vi "decode data frame.vi"(11 "字符串":string) -> (3 "EXO message":T1)   [LabVIEW 2016, in "EXO2-Sonde.lvlib"]
uses:
  EXO2-Sonde.lvlib
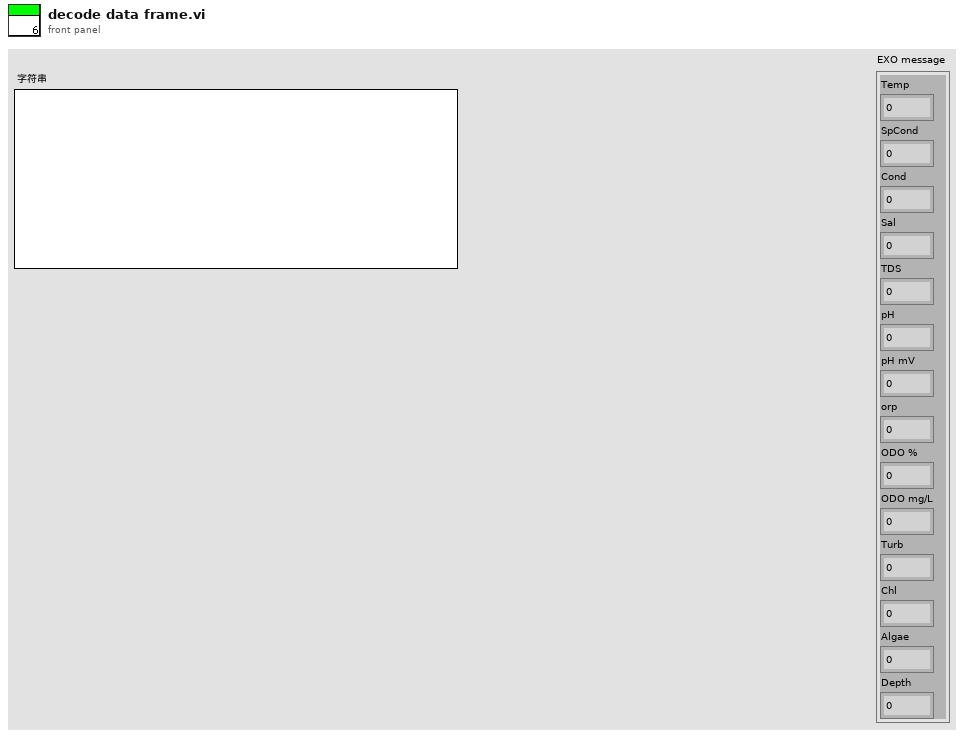
[diagram p1: front panel]
types:
  T1 = cluster{"Temp":dbl, "SpCond":dbl, "Cond":dbl, "Sal":dbl, "TDS":dbl, "pH":dbl, "pH mV":dbl, "orp":dbl, "ODO %":dbl, "ODO mg/L":dbl, "Turb":dbl, "Chl":dbl, "Algae":dbl, "Depth":dbl}
  T2 = cluster{dbl, dbl, dbl, dbl, dbl, dbl, dbl, dbl, dbl, dbl, dbl, dbl, dbl, dbl}
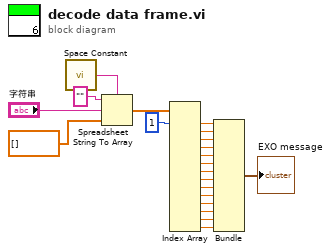
[diagram p0: block diagram]
diagram:
  n1 = call <vilib>:"Space Constant.vi"() -> ("String"=w21:string)
  n2 = Spreadsheet String To Array(delimiter (Tab)=w21, format string="" ("格式字符串"), spreadsheet string="字符串", array type (2D Dbl)=dbl[] []) -> (array=w17:dbl[])
  n3 = Index Array(array=w17, index #1=1 ("索引")) -> (element #1=w15:dbl, element #2=w3:dbl, element #3=w4:dbl, element #4=w14:dbl, element #5=w13:dbl, element #6=w12:dbl, element #7=w11:dbl, element #8=w10:dbl, element #9=w9:dbl, element #10=w8:dbl, element #11=w7:dbl, element #12=w6:dbl, element #13=w5:dbl, element #14=w1:dbl)  [unwired: 13 in]
  n4 = Bundle(w15, w3, w4, w14, w13, w12, w11, w10, w9, w8, w7, w6, w5, w1) -> (→"EXO message":T2)  [unwired: 1 in]
